vi "vision_webcam_V2_external_use_file_ref.vi"(11 "dup Message Queue 2":refnum<queue>) -> ()   [LabVIEW 2017]
uses:
  UI Error Handlers/support/Message Queue/Message Cluster.ctl
  <vilib>/userdefined/High Color/IMAQdx.ctl
  <vilib>/vision/Avi.llb/IMAQ AVI2 Refnum.ctl
  <vilib>/vision/Image Controls.llb/IMAQ Image.ctl
  Globals/Global - All RT Loop Stop.vi
  Globals/Global - Configuration Options.vi
  <vilib>/vision/driver/NI_Vision_Acquisition_Software.lvlib
  UI Error Handlers/support/Message Queue/Message Queue.lvlib
panel:
  out "appended path":path
  out "Webcam":T1(plugin-control)
  out "concatenated string 4":string
  out "error out":errorcluster
  out "x-y":u32
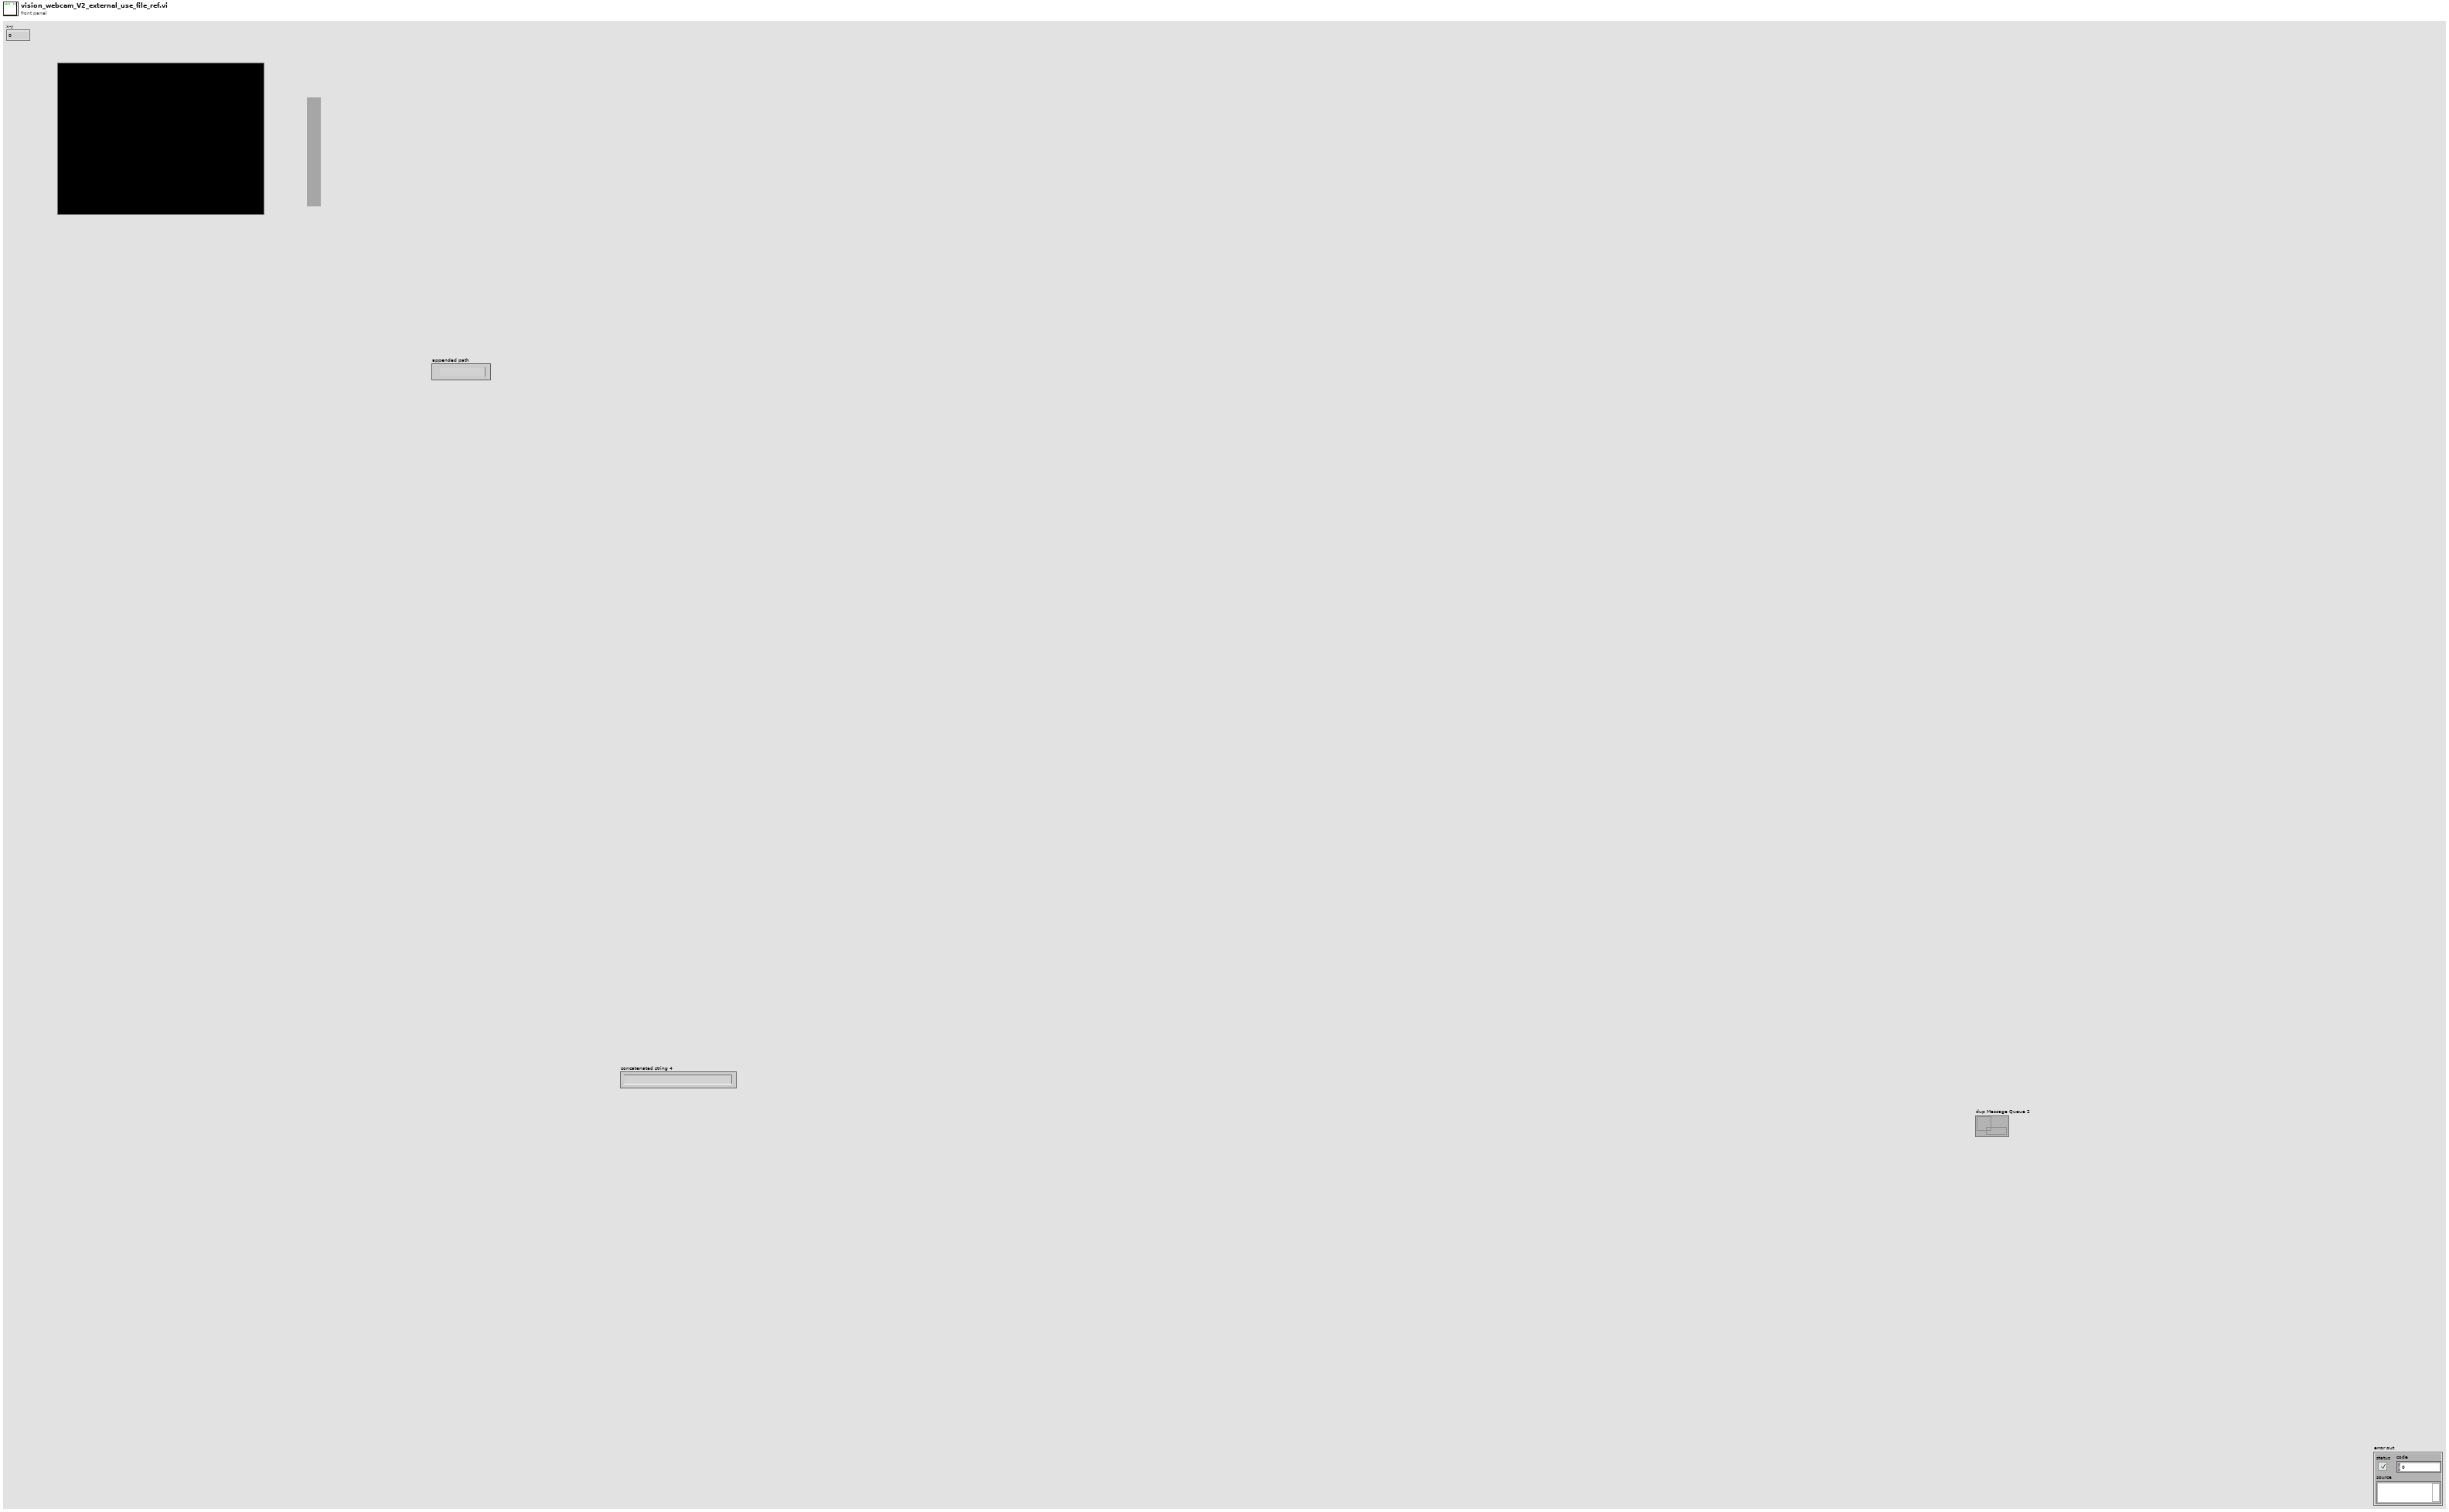
[diagram p1: front panel]
types:
  T1 = typedef "IMAQ Image.ctl" = refnum<image>
  T2 = typedef "IMAQ AVI2 Refnum.ctl" = refnum<k20>
  T3 = typedef "IMAQdx.ctl" = refnum<k21>
  T4 = typedef "Image Type" = u32
  T5 = cluster{"Tool data":cluster{"Number of teeth":sgl}, "Cutting data":cluster{"rpm":sgl}, "Limits":cluster{"Magnitude threshold":sgl, "Tolerance":sgl}, "G1 status":cluster{"G1 trigger":bool}}
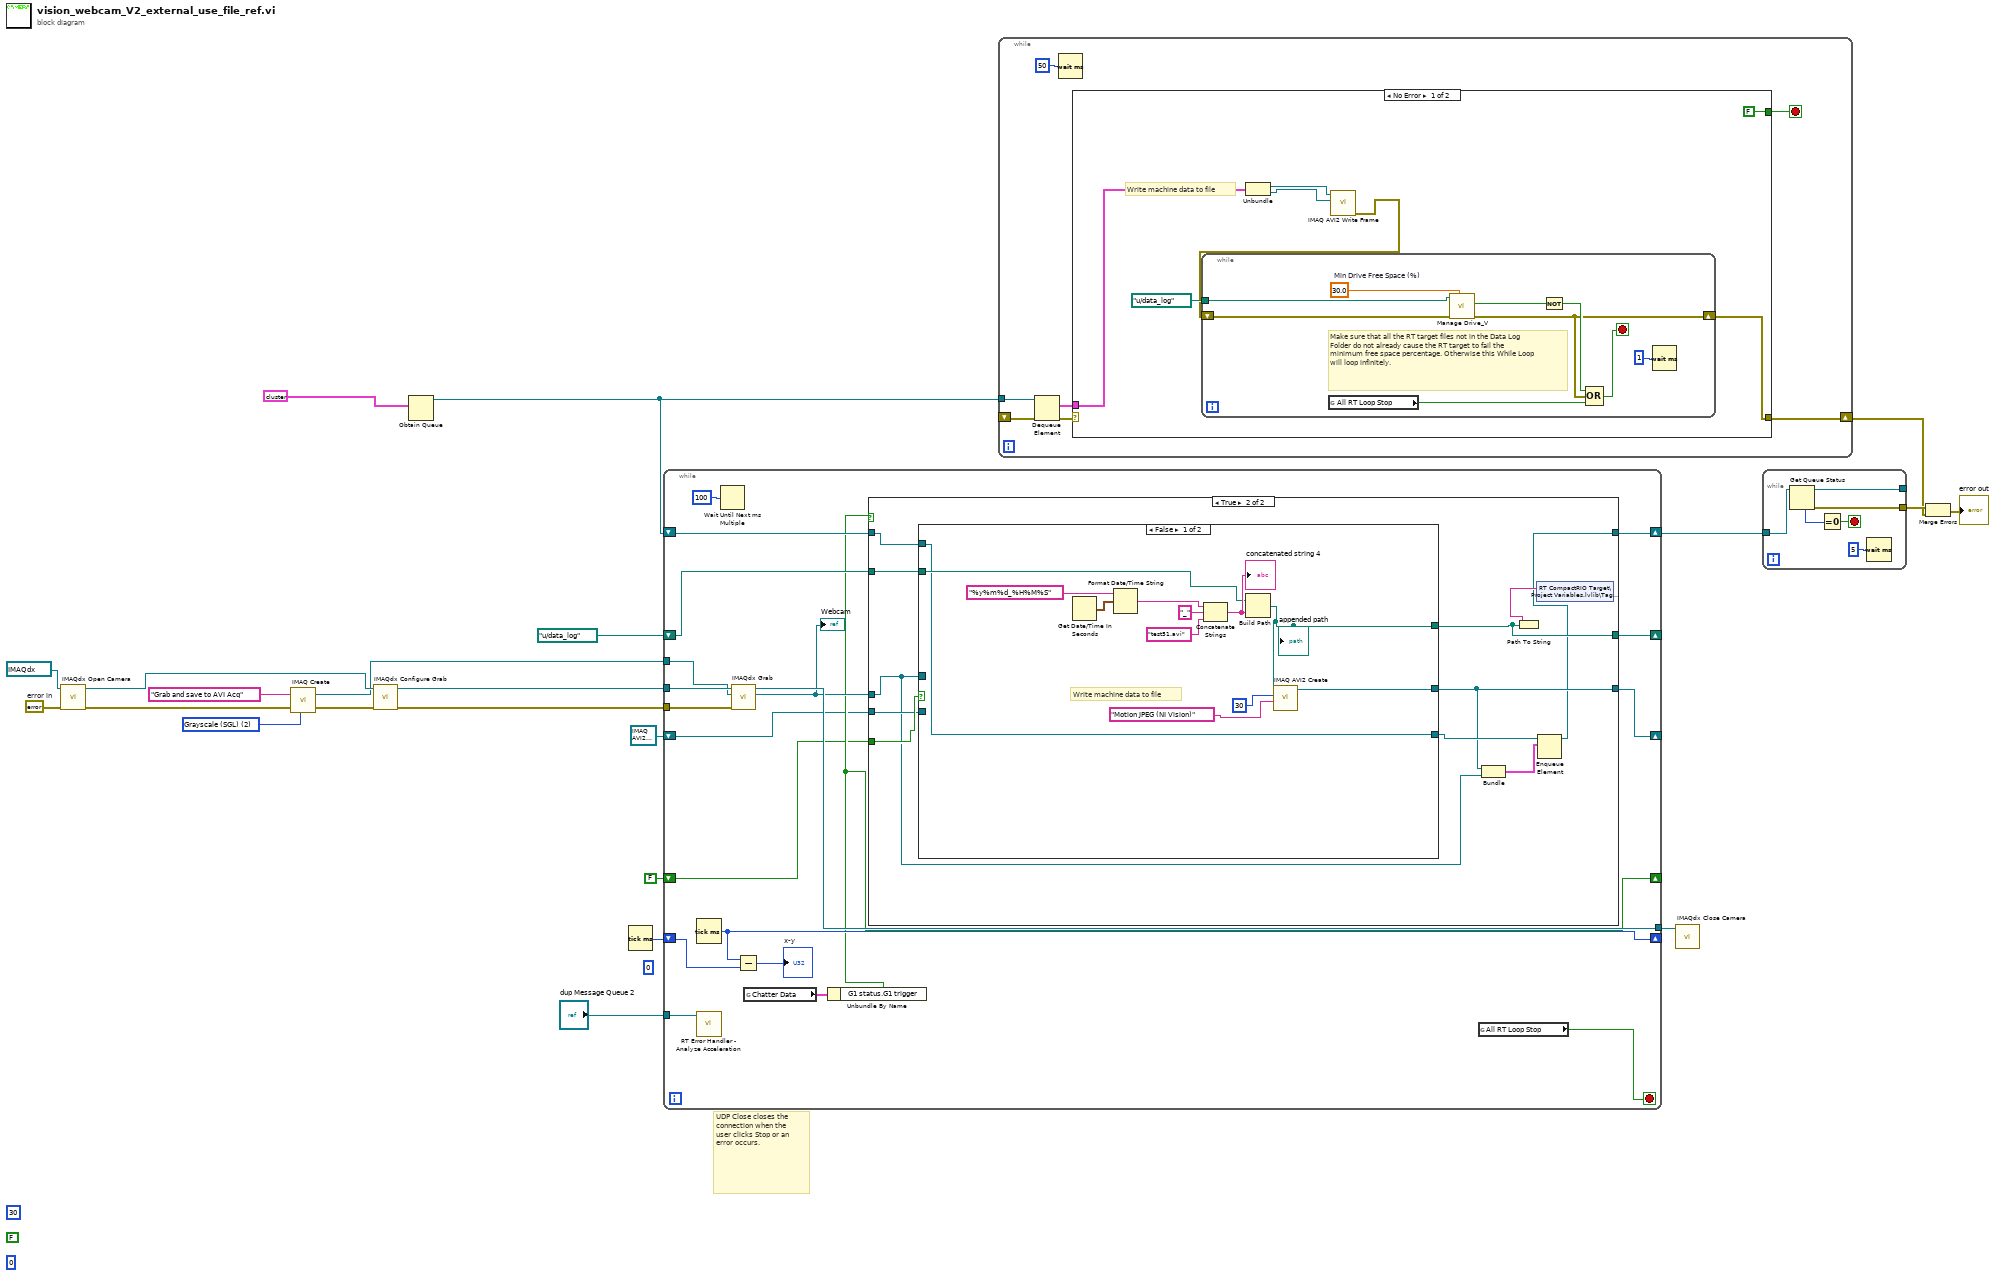
[diagram p0: block diagram]
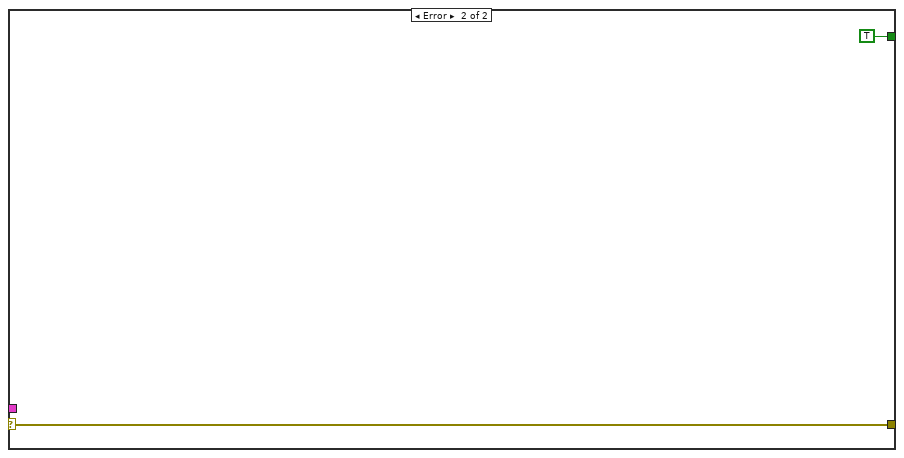
[diagram p2: hidden frame]
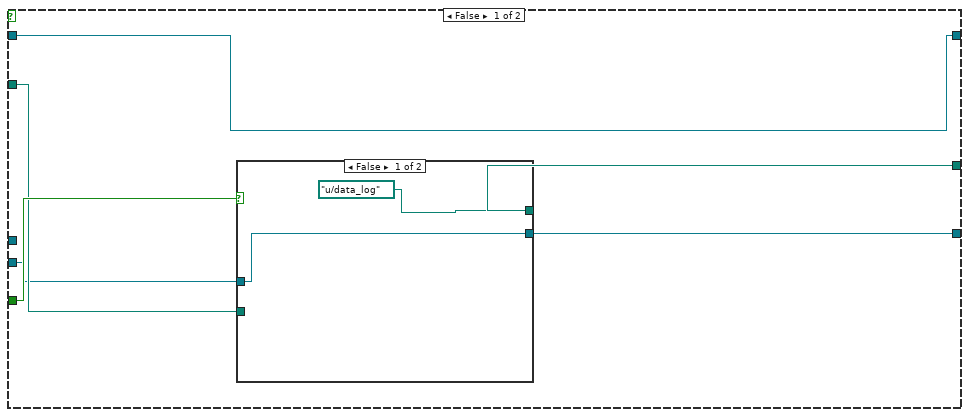
[diagram p3: hidden frame]
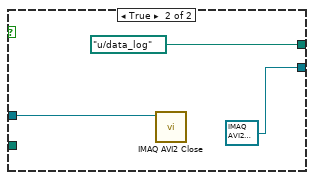
[diagram p4: hidden frame]
diagram:
  (unwired) 0
  w12 = T4 2 items=["Grayscale (U8)", "Grayscale (I16)", "Grayscale (SGL)", "Complex (CSG)", "RGB (U32)", "HSL (U32)", "RGB (U64)", "Grayscale (U16)"] ("Image Type")
  (unwired) u32 30 ("Frames Per Second")
  w13 = errorcluster {"status"=FALSE, "code"=0, "source"=""}  # error in
  (unwired) i16 0 ("A(I16) 11")
  (unwired) FALSE
  # "UDP Close closes the connection when the user clicks Stop or an error occurs."
  n1 = call <vilib>:"IMAQdx Open Camera.vi"("error in"=w13, "Session In"=T3 "cam1") -> ("error out"=w11:errorcluster, "Session Out"=w15:T3)  [unwired: 8 in]
  n2 = call "IMAQ Create"("Image Name"="Grab and save to AVI Acq", "Image Type"=w12, "error in (no error)"=w11) -> ("New Image"=w8:T1, "error out"=w7:errorcluster)  [unwired: 2 in]
  n3 = call <vilib>:"IMAQdx Configure Grab.vi"("error in"=w7, "Session In"=w15) -> ("error out"=w6:errorcluster, "Session Out"=w9:T3)  [unwired: 8 in]
  n4 = Obtain Queue(element data type=cluster{"AVI Refnum":T2, "Webcam 2":T1} {"AVI Refnum"=refnum, "Webcam 2"=refnum}) -> (queue out=w20:refnum<queue>)  [unwired: 4 in, 2 out]
  n5 = Tick Count (ms)() -> (millisecond timer value=w16:u32)
  n6 = while {
    shift-right: [w41] -> w22
    shift-left: w20 -> [w42]
    tunnel: "dup Message Queue 2" -> [w40]
    shift-right: [w36] -> _
    shift-left: w16 -> [w37]
    tunnel: w9 -> [w35]
    tunnel: w8 -> [w34]
    tunnel: w6 -> [w33]
    tunnel: [w32] -> w5
    shift-right: [w27] -> _
    shift-left: path "u:/data_log" ("AVI Path") -> [w28]
    shift-right: [w26] -> _
    shift-left: FALSE ("G1 trigger") -> [w25]
    shift-right: [w24] -> _
    shift-left: T2 refnum ("AVI Refnum") -> [w23]
    stop <- w30 stop-if-true
    n7 = Tick Count (ms)() -> (millisecond timer value=w36:u32)
    n8 = call "RT Error Handler - Analyze Acceleration.vi"("Message Queue"=w40) -> ()  [unwired: 10 in, 1 out]
    n9 = Wait Until Next ms Multiple(millisecond multiple=u32 100) -> ()  [unwired: 1 out]
    n10 = call <vilib>:"IMAQdx Grab.vi"("error in"=w33, "Image In"=w34, "Session In"=w35) -> ("Image Out"=w29:T1, "Session Out"=w32:T3)  [unwired: 5 in, 2 out]
    "Webcam" <- w29
    n11 = Subtract(x=w36, y=w37) -> (x-y=→"x-y":u32)
    n12 = global read "Global - Configuration Options.vi" "Chatter Data"() -> (w39:T5)
    n13 = Unbundle By Name(w39) -> ("G1 status.G1 trigger"=w26:bool)
    n14 = case shown="True" w26 {
      tunnel: w42 -> [w43 w60]
      tunnel: [w43 w54] -> w41
      tunnel: w29 -> [_ w56]
      tunnel: w28 -> [w46 w63]
      tunnel: [w48 w62] -> w27
      tunnel: w25 -> [w47 w61]
      tunnel: [w44 w55] -> w24
      tunnel: w23 -> [w45 w59]
      frame False {
        n15 = case shown="False" w47 {
          tunnel: [path "u:/data_log" ("AVI Path") path "u:/data_log" ("AVI Path")] -> w48
          tunnel: w46 -> [_ _]
          tunnel: w45 -> [w49 w52]
          tunnel: [w49 T2 refnum ("AVI Refnum")] -> w44
          frame False {
          }
          frame True {
            n16 = call "IMAQ AVI2 Close"("AVI Refnum"=w52) -> ()  [unwired: 10 in, 1 out]
          }
        }
      }
      frame True {
        n17 = case shown="False" w61 {
          tunnel: w56 -> [_ _]
          tunnel: w60 -> [w69 w78]
          tunnel: [w66 w79] -> w62
          tunnel: w63 -> [w70 w79]
          tunnel: [w69 w78] -> w58
          tunnel: [w65 w77] -> w55
          tunnel: w59 -> [_ w77]
          frame False {
            # "Write machine data to file"
            n18 = Get Date/Time In Seconds() -> (seconds since 1Jan1904=w74:timestamp)
            n19 = Format Date/Time String(time format string (%c)="%y%m%d_%H%M%S", seconds (now)=w74) -> (date/time string=w75:string)  [unwired: 1 out]
            n20 = Concatenate Strings(w75, "_" ("string"), "test51.avi" ("name or relative path")) -> (w76:string)
            "concatenated string 4" <- w76
            n21 = Build Path(base path=w70, name or relative path=w76) -> (appended path=w66:path)
            "appended path" <- w66
            n22 = call "IMAQ AVI2 Create"("Codec"="Motion JPEG (NI Vision)", "Frames Per Second"=u32 30, "AVI Path"=w66) -> ("AVI Refnum"=w65:T2)  [unwired: 7 in, 1 out]
          }
          frame True {
          }
        }
        n23 = Bundle("AVI Refnum"=w55, "Image Out"=w56) -> (w57:cluster{"AVI Refnum":T2, "Image Out":T1})  [unwired: 1 in]
        n24 = Path To String(path=w62) -> (string=w64:string)
        n25 = shared-variable "RT CompactRIO Target\\Project Variables.lvlib\\Tag Video"(w64) -> ()  [unwired: 1 in, 1 out]
        n26 = Enqueue Element(queue=w58, element=w57) -> (queue out=w54:refnum<queue>)  [unwired: 2 in, 2 out]
      }
    }
    n27 = global read "Global - All RT Loop Stop.vi" "All RT Loop Stop"() -> (w30:bool)
  }
  n28 = while {
    tunnel: w20 -> [w86]
    shift-right: [w82] -> w19
    shift-left: _ -> [w85]
    stop <- w83 stop-if-true
    n29 = Dequeue Element(queue=w86, error in (no error)=w85) -> (element=w81:cluster{"AVI Refnum":T2, "Webcam 2":T1}, error out=w84:errorcluster)  [unwired: 1 in, 2 out]
    n30 = Wait (ms)(milliseconds to wait=u32 50) -> ()  [unwired: 1 out]
    n31 = case shown="No Error" w84 {
      selector: w84 -> [_ w103]
      tunnel: [FALSE TRUE] -> w83
      tunnel: [w91 w103] -> w82
      tunnel: w81 -> [w90 _]
      frame No Error {
        # "Write machine data to file"
        n32 = Unbundle(w90) -> ("AVI Refnum"=w88:T2, "Webcam 2"=w87:T1)
        n33 = call "IMAQ AVI2 Write Frame"("Image"=w87, "AVI Refnum"=w88) -> ("error out"=w89:errorcluster)  [unwired: 7 in, 2 out]
        n34 = while {
          shift-right: [w97] -> w91
          shift-left: w89 -> [w98]
          tunnel: path "u:/data_log" ("AVI Path") -> [w95]
          stop <- w102 stop-if-true
          w96 = 30.0  # Min Drive Free Space (%)
          # "Make sure that all the RT target files not in the Data Log Folder do not already cause the RT target to fail the minimum free space percentage. Otherwise this While Loop will loop infinitely."
          n35 = global read "Global - All RT Loop Stop.vi" "All RT Loop Stop"() -> (w99:bool)
          n36 = call "Manage Drive_V.vi"("Min Drive Free Space (%)"=w96, "error in"=w98, "Data Folder"=w95) -> ("error out"=w97:errorcluster, "Drive Space Below Limit"=w94:bool)  [unwired: 6 in, 1 out]
          n37 = Not(x=w94) -> (.not. x?=w101:bool)
          n38 = Compound Arithmetic op=OR(w101, w97, w99) -> (w102:bool)
          n39 = Wait (ms)(milliseconds to wait=u32 1) -> ()  [unwired: 1 out]
        }
      }
      frame Error {
      }
    }
  }
  n40 = call <vilib>:"IMAQdx Close Camera.vi"("Session In"=w5) -> ()  [unwired: 10 in, 1 out]
  n41 = while {
    tunnel: [w109] -> w21
    tunnel: [w107] -> _
    tunnel: w22 -> [w105]
    stop <- w108 stop-if-true
    n42 = Get Queue Status(queue=w105) -> (queue out=w107:refnum<queue>, error out=w109:errorcluster, # elements in queue=w106:i32)  [unwired: 2 in, 5 out]
    n43 = Equal To 0?(x=w106) -> (x = 0?=w108:bool)
    n44 = Wait (ms)(milliseconds to wait=u32 5) -> ()  [unwired: 1 out]
  }
  n45 = Merge Errors(w21, w19) -> (→"error out":errorcluster)
